vi "Init Processing.vi"(11 "Processing In":refnum<class "Processing.lvclass">) -> (3 "Processing":refnum<class "Processing.lvclass">)   [LabVIEW 2020, in "HTTP Server.lvlib" / "Server.lvclass"]
uses:
  Server.lvclass
  Processing/Processing.lvclass
  Security/Security.lvclass
  C:/dev/lv20CE/relink/lv-http-server/HTTP Server/Service/Service.lvclass
  Processing/Processing.lvclass/Processing.ctl
  Server.lvclass/Server.ctl
  Values/Values.lvclass
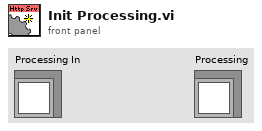
[diagram p1: front panel]
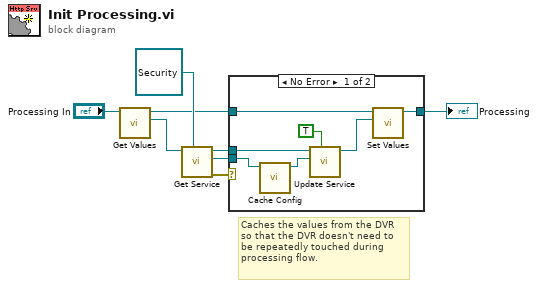
[diagram p0: block diagram]
diagram:
  # "Caches the values from the DVR so that the DVR doesn't need to be repeatedly touched during processing flow."
  n1 = call "Get Values.vi"("Processing in"="Processing In") -> ("Values"=w4:refnum<class "Values.lvclass">, "Processing out"=w3:refnum<class "Processing.lvclass">)  [unwired: 9 in]
  n2 = call "Get Service.vi"("Service Type"=refnum<class "Security.lvclass"> refnum ("HTTP Server.lvlib:Security.lvclass"), "Values in"=w4) -> ("error out"=w1:errorcluster, "Service"=w7:refnum<class "Security.lvclass">, "Values out"=w6:refnum<class "Values.lvclass">)  [unwired: 7 in]
  n3 = case shown="No Error" w1 {
    tunnel: w7 -> [w15 _]
    tunnel: w6 -> [w14 _]
    tunnel: w3 -> [w11 w16]
    tunnel: [w10 w16] -> w2
    frame No Error {
      n4 = call "Cache Config.vi"("Security in"=w15) -> ("Security out"=w12:refnum<class "Security.lvclass">)  [unwired: 9 in, 1 out]
      n5 = call "Update Service.vi"("Overwrite? (F)"=TRUE, "Service"=w12, "Values in"=w14) -> ("Values out"=w9:refnum<class "Values.lvclass">)  [unwired: 7 in, 1 out]
      n6 = call "Set Values.vi"("Values"=w9, "Processing in"=w11) -> ("Processing out"=w10:refnum<class "Processing.lvclass">)  [unwired: 9 in]
    }
    frame Error {
      # "Security is not enabled, do nothing."
    }
  }
  "Processing" <- w2
